vi "DeLinkFixFromSerialNumber.vi"(0 "class data in":refnum<class "CMESAPI.lvclass">, 5 "serialNumber":string, 11 "error in (no error)":errorcluster) -> (4 "class data out":refnum<class "CMESAPI.lvclass">, 6 "DeLinkFixtureFromSerialNumber":string, 15 "error out":errorcluster)   [LabVIEW 2020, in "Salcomp-MES.lvlib" / "CMESAPI.lvclass"]
uses:
  CMESAPI.lvclass
  CMESAPI.lvclass/CMESAPI.ctl
  E:/Git/Libraries/develop/CME-API/CMESAPI_Fw4.0_1.9.2/CMESAPI.dll
  CMESAPI_Fw4.0_1.9.2/CMESAPI.dll
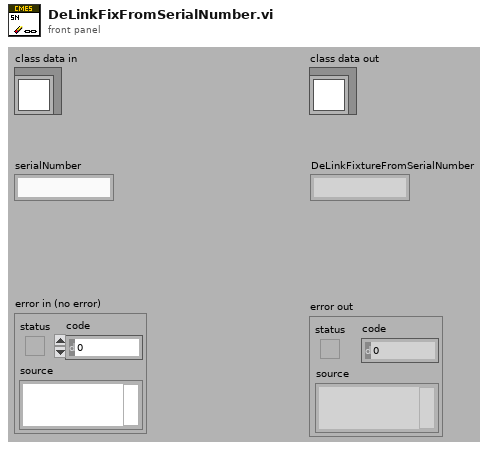
[diagram p1: front panel]
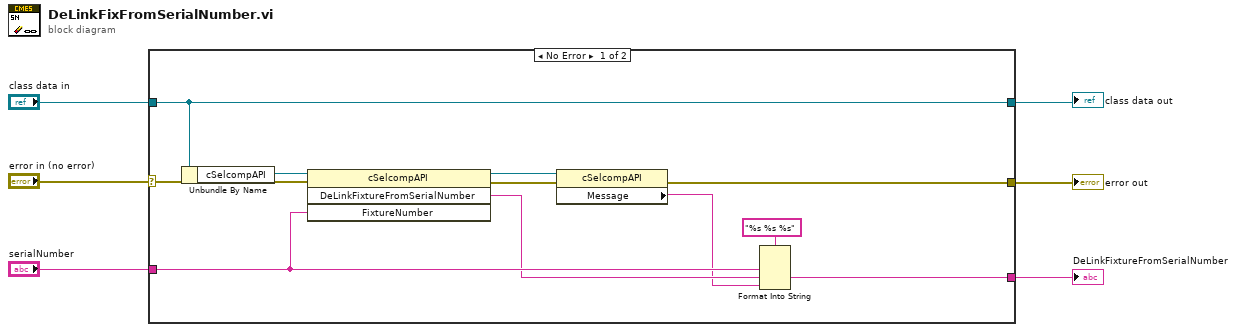
[diagram p0: block diagram]
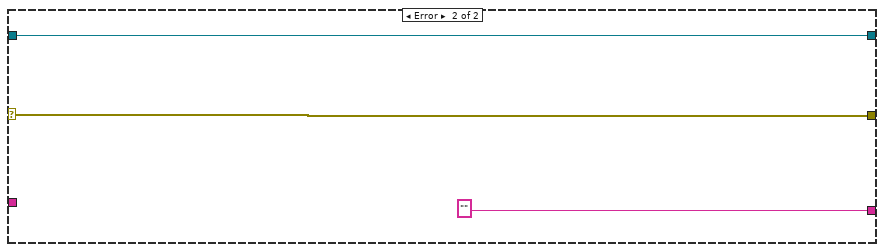
[diagram p2: hidden frame]
diagram:
  n1 = case shown="No Error" "error in (no error)" {
    selector: "error in (no error)" -> [w14 w19]
    tunnel: [w10 w19] -> w5
    tunnel: "class data in" -> [w16 w18]
    tunnel: [w16 w18] -> w3
    tunnel: "serialNumber" -> [w9 _]
    tunnel: [w8 "" ("DeLinkFixtureFromSerialNumber")] -> w1
    frame No Error {
      n2 = Unbundle By Name(w16) -> ("cSelcompAPI"=w15:refnum<k24>)
      n3 = invoke on="Invoke Node" class="cSelcompAPI" method="DeLinkFixtureFromSerialNumber"(reference=w15, error in=w14, "FixtureNumber"=w9) -> (reference out=w12:refnum<k24>, error out=w13:errorcluster, "DeLinkFixtureFromSerialNumber"=w8:string)  [unwired: 1 in, 1 out]
      n4 = property class="cSelcompAPI"(reference=w12, error in=w13) -> (error out=w10:errorcluster, "Message"=w7:string)  [unwired: 1 out]
      n5 = Format Into String(format string="%s %s %s", w9, w8, w7) -> ()  [unwired: 2 in, 2 out]
    }
    frame Error {
    }
  }
  "error out" <- w5
  "class data out" <- w3
  "DeLinkFixtureFromSerialNumber" <- w1
